vi "Write Notifier Map.vi"(8 "error in (no error)":errorcluster, 10 "Notifier Map":map{i64, refnum<class "Notifier.lvclass">}(c390), 11 "Simiple Map SEQ 64 Notifier Controller Factory in":refnum<class "Simiple Map Notifier Controller Factory.lvclass">) -> (0 "error out":errorcluster, 3 "Simiple Map SEQ 64 Notifier Controller Factory out":refnum<class "Simiple Map Notifier Controller Factory.lvclass">)   [LabVIEW 2024, in "Simiple Map Notifier Controller Factory.lvclass"]
uses:
  Simiple Map Notifier Controller Factory.lvclass
  Ancestor Class/Actor Assistant/Notifier/Notifier.lvclass
  Simiple Map Notifier Controller Factory.lvclass/Simiple Map Notifier Controller Factory.ctl
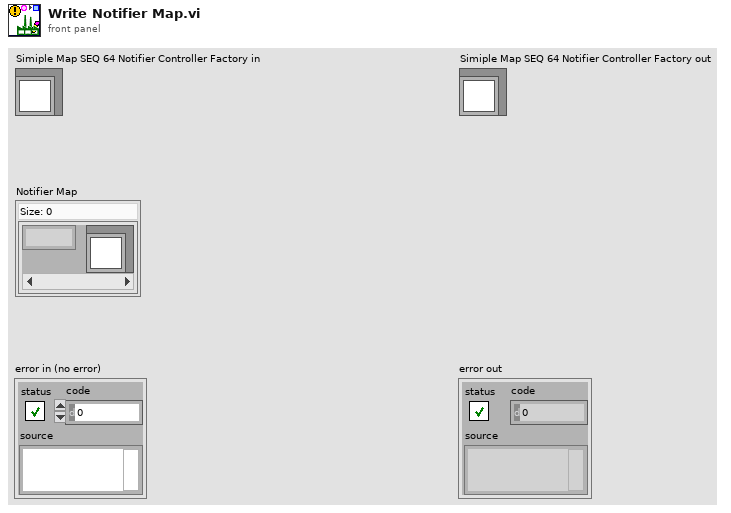
[diagram p1: front panel]
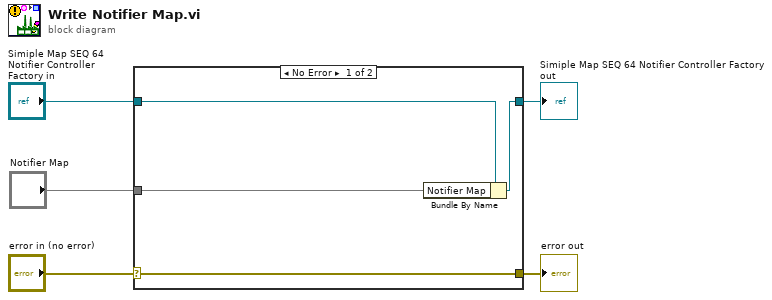
[diagram p0: block diagram]
diagram:
  n1 = case shown="No Error" "error in (no error)" {
    selector: "error in (no error)" -> [w9 w10]
    tunnel: [w9 w10] -> w4
    tunnel: [w7 w11] -> w2
    tunnel: "Simiple Map SEQ 64 Notifier Controller Factory in" -> [w8 w11]
    tunnel: "Notifier Map" -> [w6 _]
    frame No Error {
      n2 = Bundle By Name(cluster=w8, "Notifier Map"=w6) -> (w7:refnum<class "Simiple Map Notifier Controller Factory.lvclass">)
    }
    frame Error {
    }
  }
  "error out" <- w4
  "Simiple Map SEQ 64 Notifier Controller Factory out" <- w2
